vi "_ROSMasterConsole.vi"() -> ()   [LabVIEW 2010]
uses:
  <vilib>/Utility/miscctls.llb/LVRectTypeDef.ctl
  <userlib>/ROSforLV_0.1/ROS/Code/_ROSDefinition.vi
panel:
  in  "Clear Servers?":bool
  in  "expand?":bool
  out "Status":string
  out "Master?":bool
  in  "Tab Control":enum32{"Single Calls", "Servers"}(tab)
  out "TCP Calls":T1(array[cluster])
  out "ROS Master":string="192.168.1.110:11311"
  out "Running?":bool
  out "current task":string
  in  "Stop":bool
  in  "Live Servers":i32(listbox)
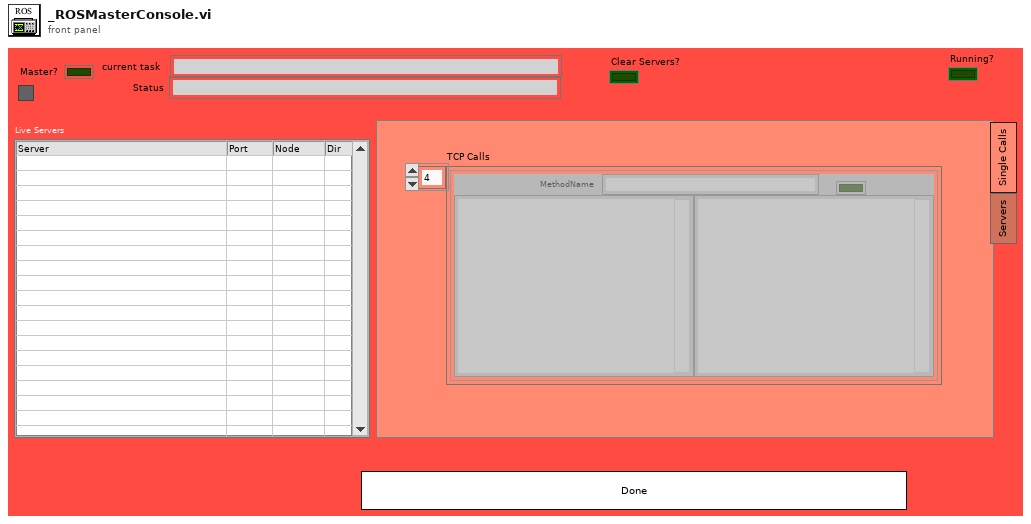
[diagram p1: front panel]
types:
  T1 = cluster{"First":string, "Second":string, "MethodName":string, "success":bool, "Dir1":string, "Dir2":string}[]
  T2 = cluster{"server vi":string, "reference":refnum<vi>, "Description":string[]}[]
  T3 = cluster{"Request":string, "Reply":string, "MethodName":string, "success":bool, "Request 2":string, "Request 3":string}[]
  T4 = cluster{"Request":string, "Reply":string, "MethodName":string, "success":bool, "first string":string, "second string":string}
  T5 = typedef "LVRectTypeDef.ctl" = cluster{"Left":i16, "Top":i16, "Right":i16, "Bottom":i16}
  T6 = typedef "_ROSControl.ctl" = cluster{"topic port":u16, "Node":string, "topic":string, "type":string, "node port":u32, "error ":errorcluster, "Direction":T7, "APIs":string[]}
  T7 = typedef "_ROSDirection.ctl" = enum16{"Node", "Publisher", "Subscriber", "Service Client"}
  T8 = cluster{"server vi":string, "reference":refnum<vi>, "Description":string[]}
  T9 = cluster{"data out":string, "data out 2":string, "data out 3":string, "Success?":bool, "data out 4":string, "data out 5":string}[]
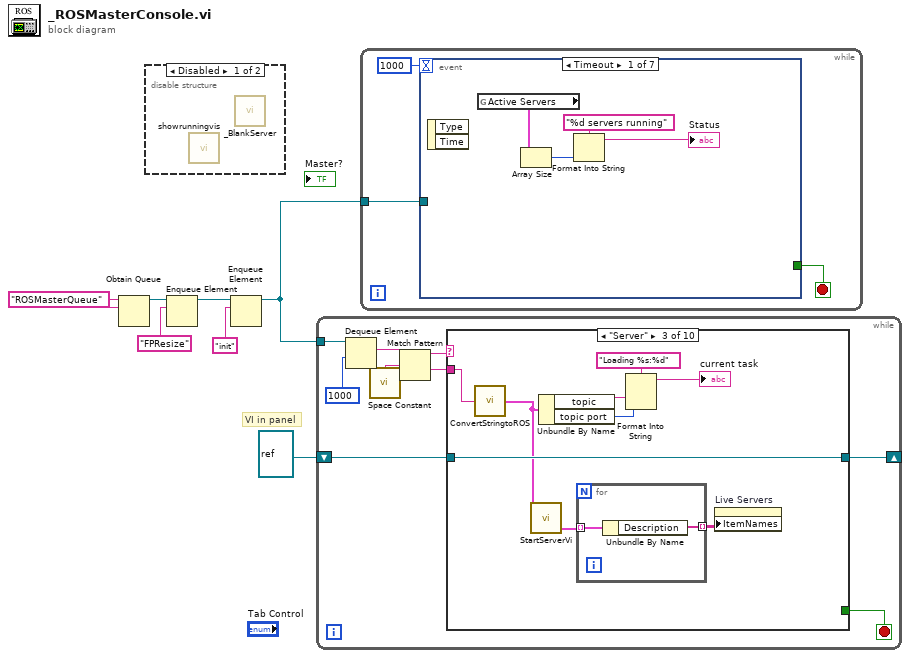
[diagram p0: block diagram]
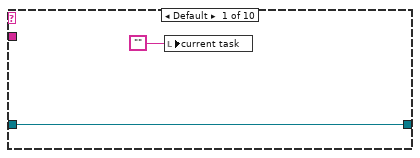
[diagram p3: hidden frame]
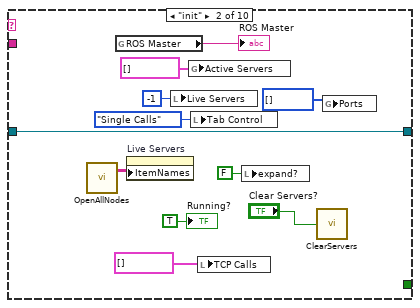
[diagram p4: hidden frame]
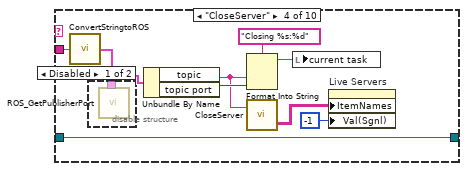
[diagram p5: hidden frame]
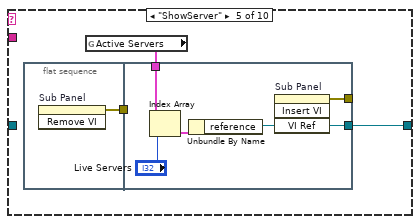
[diagram p7: hidden frame]
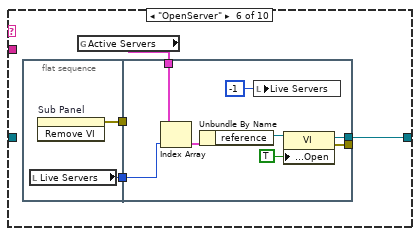
[diagram p8: hidden frame]
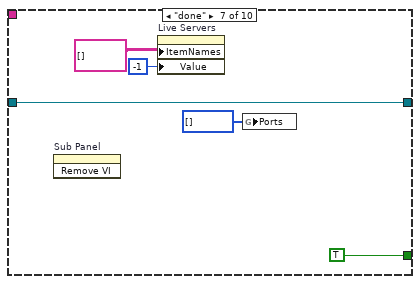
[diagram p9: hidden frame]
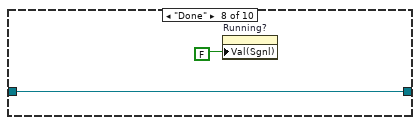
[diagram p10: hidden frame]
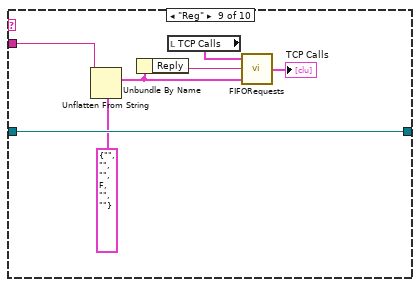
[diagram p11: hidden frame]
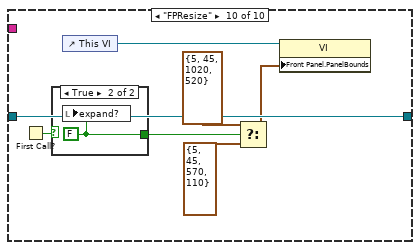
[diagram p12: hidden frame]
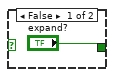
[diagram p13: hidden frame]
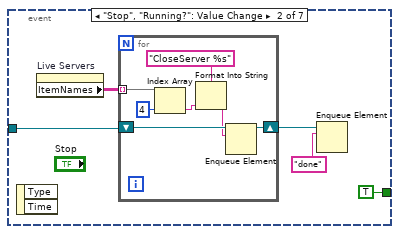
[diagram p14: hidden frame]
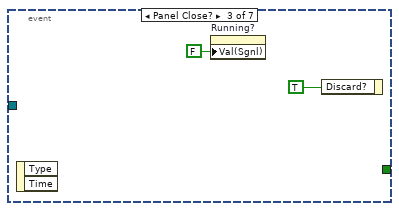
[diagram p15: hidden frame]
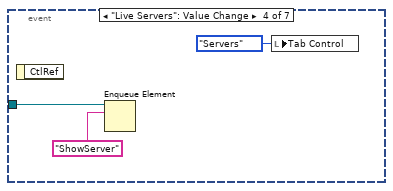
[diagram p16: hidden frame]
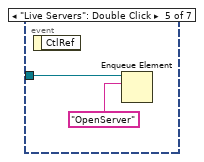
[diagram p17: hidden frame]
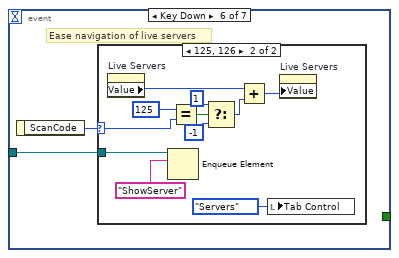
[diagram p18: hidden frame]
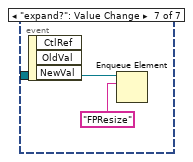
[diagram p20: hidden frame]
diagram:
  w7 = "ROSMasterQueue" ("name (unnamed)")
  # "VI in panel"
  n1 = Obtain Queue(name (unnamed)=w7, element data type=w7) -> (queue out=w4:refnum<queue>)  [unwired: 3 in, 2 out]
  n2 = disable-structure shown="Disabled" {
    frame Disabled {
      n3 = call <userlib>:"showrunningvis.vi"() -> ()  [unwired: 1 in]
      n4 = call <userlib>:"_BlankServer.vi"() -> ()  [unwired: 12 in]
    }
    frame Enabled {
    }
  }
  n5 = Enqueue Element(queue=w4, element="FPResize") -> (queue out=w3:refnum<queue>)  [unwired: 2 in, 2 out]
  n6 = Enqueue Element(queue=w3, element="init") -> (queue out=w6:refnum<queue>)  [unwired: 2 in, 2 out]
  n7 = while {
    tunnel: w6 -> [w16]
    shift-right: [w9] -> _
    shift-left: refnum<vi> refnum ("VI Ref") -> [w10]
    stop <- w15 stop-if-true
    n8 = Dequeue Element(queue=w16, timeout in ms (-1)=1000) -> (element=w13:string)  [unwired: 1 in, 3 out]
    n9 = call <vilib>:"Space Constant.vi"() -> ("String"=w12:string)
    n10 = Match Pattern(string=w13, regular expression=w12) -> (before substring=w14:string, after substring=w11:string)  [unwired: 1 in, 2 out]
    n11 = case shown="\"Server\"" w14 {
      tunnel: [_ _ _ _ _ _ TRUE _ _ _] -> w15
      tunnel: w11 -> [_ _ w35 w44 _ _ _ _ w86 _]
      tunnel: w10 -> [w18 w29 w38 w49 _ _ w77 w80 w87 w94]
      tunnel: [w18 w29 w38 w49 w51 w60 w77 w80 w87 w94] -> w9
      frame Default {
        n12 = local write "current task"("") -> ()
      }
      frame "init" {
        n13 = call <userlib>:"OpenAllNodes.vi"() -> ("Nodes"=w27:string[][])  [unwired: 2 in]
        n14 = global read "_ROSDefinition.vi" "ROS Master"() -> (→"ROS Master":string)
        n15 = property on="Live Servers" class="MCListbox (strict)"("ItemNames"=w27) -> ()  [unwired: 2 in, 2 out]
        n16 = local write "Live Servers"(-1 ("Live Servers")) -> ()
        n17 = global write "_ROSDefinition.vi" "Active Servers"(T2 [] ("Active Servers")) -> ()
        n18 = local write "Tab Control"(enum32{"Single Calls", "Servers"}."Single Calls" ("Tab Control")) -> ()
        n19 = local write "TCP Calls"(T3 [] ("TCP Calls")) -> ()
        n20 = local write "expand?"(FALSE ("expand?")) -> ()
        n21 = call <userlib>:"ClearServers.vi"("Clear Servers?"="Clear Servers?") -> ()  [unwired: 1 out]
        n22 = global write "_ROSDefinition.vi" "Ports"(u16[] [] ("Ports")) -> ()
        "Running?" <- TRUE ("Running?")
      }
      frame "Server" {
        n23 = call <userlib>:"ConvertStringtoROS.vi"("string in"=w35) -> ("ROS"=w31:T6)
        n24 = call <userlib>:"StartServerVi.vi"("Baxter"=w31) -> ("Active Topics"=w32:T2)  [unwired: 2 out]
        n25 = Unbundle By Name(w31) -> ("topic"=w34:string, "topic port"=w33:u16)
        n26 = for {
          tunnel: w32 -> [w40] mode=indexing
          tunnel: [w39] -> w30 mode=indexing
          n27 = Unbundle By Name(w40) -> ("Description"=w39:string[])
        }
        n28 = Format Into String(format string="Loading %s:%d", w34, w33) -> (resulting string=→"current task":string)  [unwired: 2 in, 1 out]
        n29 = property on="Live Servers" class="MCListbox (strict)"("ItemNames"=w30) -> ()  [unwired: 2 in, 2 out]
      }
      frame "CloseServer" {
        n30 = call <userlib>:"ConvertStringtoROS.vi"("string in"=w44) -> ("ROS"=w41:T6)
        n31 = disable-structure shown="Disabled" {
          disable-tunnel: w41 -> [w50 _]
          frame Disabled {
            n32 = call <userlib>:"ROS_GetPublisherPort.vi"("ROS in"=w50) -> ()  [unwired: 1 in, 2 out]
          }
          frame Enabled {
          }
        }
        n33 = Unbundle By Name(w41) -> ("topic"=w42:string, "topic port"=w43:u16)
        n34 = Format Into String(format string="Closing %s:%d", w42, w43) -> (resulting string=w47:string)  [unwired: 2 in, 1 out]
        n35 = call <userlib>:"CloseServer.vi"("Server"=w42) -> ("Active Servers Out"=w46:string[][])  [unwired: 2 in]
        n36 = local write "current task"(w47) -> ()
        n37 = property on="Live Servers" class="MCListbox (strict)"("ItemNames"=w46, "Val(Sgnl)"=-1 ("Value (Signaling)")) -> ()  [unwired: 2 in, 2 out]
      }
      frame "ShowServer" {
        n38 = flat-sequence {
          tunnel: [w54] -> w53
          tunnel: w53 -> [_]
          tunnel: [w58] -> _
          tunnel: w52 -> [w57]
          tunnel: [w55] -> w51
          frame #0 {
            n39 = invoke on="Sub Panel" class="SubPanel" method="Remove VI"() -> (error out=w54:errorcluster)  [unwired: 3 in, 2 out]
          }
          frame #1 {
            n40 = Index Array(array=w57, index="Live Servers") -> (element=w56:T8)
            n41 = Unbundle By Name(w56) -> ("reference"=w55:refnum<vi>)
            n42 = invoke on="Sub Panel" class="SubPanel" method="Insert VI"("VI Ref"=w55) -> (error out=w58:errorcluster)  [unwired: 3 in, 3 out]
          }
        }
        n43 = global read "_ROSDefinition.vi" "Active Servers"() -> (w52:T2)
      }
      frame "OpenServer" {
        n44 = flat-sequence {
          tunnel: [w65] -> w63
          tunnel: [w64] -> w62
          tunnel: w63 -> [_]
          tunnel: w62 -> [w72]
          tunnel: w61 -> [w70]
          tunnel: [w67] -> w60
          tunnel: [w66] -> _
          frame #0 {
            n45 = local read "Live Servers"() -> (w64:i32)
            n46 = invoke on="Sub Panel" class="SubPanel" method="Remove VI"() -> (error out=w65:errorcluster)  [unwired: 3 in, 2 out]
          }
          frame #1 {
            n47 = Index Array(array=w70, index=w72) -> (element=w69:T8)
            n48 = Unbundle By Name(w69) -> ("reference"=w68:refnum<vi>)
            n49 = local write "Live Servers"(-1 ("Live Servers")) -> ()
            n50 = property class="VI"(reference=w68, "Front Panel.Open"=TRUE ("Front Panel Window:Open")) -> (reference out=w67:refnum<vi>, error out=w66:errorcluster)  [unwired: 1 in]
          }
        }
        n51 = global read "_ROSDefinition.vi" "Active Servers"() -> (w61:T2)
      }
      frame "done" {
        n52 = invoke on="Sub Panel" class="SubPanel" method="Remove VI"() -> ()  [unwired: 3 in, 3 out]
        n53 = property on="Live Servers" class="MCListbox (strict)"("ItemNames"=string[][] [] ("Item Names"), "Value"=-1 ("Live Servers")) -> ()  [unwired: 2 in, 2 out]
        n54 = global write "_ROSDefinition.vi" "Ports"(u16[] [] ("Ports")) -> ()
      }
      frame "Done" {
        n55 = property on="Running?" class="Bool (strict)"("Val(Sgnl)"=FALSE) -> ()  [unwired: 2 in, 2 out]
      }
      frame "Reg" {
        n56 = Unflatten From String(type=T4 {"Request"="", "Reply"="", "MethodName"="", "success"=FALSE, "first string"="", "second string"=""} ("Reg"), binary string=w86) -> (value=w82:T4)  [unwired: 3 in, 2 out]
        n57 = Unbundle By Name(w82) -> ("Reply"=w81:string)
        n58 = local read "TCP Calls"() -> (w84:T1)
        n59 = call <userlib>:"FIFORequests.vi"("New One"=w82, "data out"=w81, "Requests In"=w84) -> ("Requests Out"=→"TCP Calls":T9)
      }
      frame "FPResize" {
        n60 = First Call?() -> (First Call?: T/F=w89:bool)
        n61 = case shown="True" w89 {
          tunnel: ["expand?" w96] -> w88
          frame False {
          }
          frame True {
            w96 = FALSE ("expand?")
            n62 = local write "expand?"(w96) -> ()
          }
        }
        n63 = control-ref of="This VI"() -> (w93:refnum<vi>)
        n64 = Select(t=T5 {"Left"=5, "Top"=45, "Right"=1020, "Bottom"=520} ("Front Panel Window:Panel Bounds"), s=w88, f=T5 {"Left"=5, "Top"=45, "Right"=570, "Bottom"=110} ("Front Panel Window:Panel Bounds")) -> (s? t:f=w91:T5)
        n65 = property class="VI"(reference=w93, "Front Panel.PanelBounds"=w91) -> ()  [unwired: 1 in, 2 out]
      }
    }
  }
  n66 = while {
    tunnel: w6 -> [w99]
    stop <- w98 stop-if-true
    n67 = event shown="[0] Timeout" {
      selector: _ -> [_ _ _ _ _ _ _]
      dyn-events: _ -> [_ _ _ _ _ _ _]
      timeout: 1000 -> [_ _ _ _ _ _ _]
      tunnel: w99 -> [_ w106 _ w119 w121 w124 w136]
      tunnel: [_ TRUE ("Stop") _ _ _ _ _] -> w98
      event Timeout {
        n68 = event-data() -> ()  [unwired: 1 in, 2 out]
        n69 = global read "_ROSDefinition.vi" "Active Servers"() -> (w100:T2)
        n70 = Array Size(array=w100) -> (size(s)=w103:i32)
        n71 = Format Into String(format string="%d servers running", w103) -> (resulting string=→"Status":string)  [unwired: 2 in, 1 out]
      }
      event "Stop", "Running?": Value Change {
        n72 = event-data() -> ()  [unwired: 1 in, 2 out]
        n73 = property on="Live Servers" class="MCListbox (strict)"() -> ("ItemNames"=w107:string[][])  [unwired: 2 in, 2 out]
        n74 = for {
          tunnel: w107 -> [w115] mode=indexing
          shift-right: [w109] -> w105
          shift-left: w106 -> [w111]
          n75 = Index Array(array=w115, index=4) -> (element=w113:string)
          n76 = Format Into String(format string="CloseServer %s", w113) -> (resulting string=w110:string)  [unwired: 2 in, 1 out]
          n77 = Enqueue Element(queue=w111, element=w110) -> (queue out=w109:refnum<queue>)  [unwired: 2 in, 2 out]
        }
        n78 = Enqueue Element(queue=w105, element="done") -> ()  [unwired: 2 in, 3 out]
      }
      event Panel Close? {
        n79 = event-data() -> ()  [unwired: 1 in, 2 out]
        n80 = property on="Running?" class="Bool (strict)"("Val(Sgnl)"=FALSE ("Value (Signaling)")) -> ()  [unwired: 2 in, 2 out]
        n81 = event-data("Discard?"=TRUE ("Stop")) -> ()  [unwired: 1 in, 1 out]
      }
      event "Live Servers": Value Change {
        n82 = event-data() -> ()  [unwired: 1 in, 1 out]
        n83 = Enqueue Element(queue=w119, element="ShowServer") -> ()  [unwired: 2 in, 3 out]
        n84 = local write "Tab Control"(enum32{"Single Calls", "Servers"}."Servers" ("Tab Control")) -> ()
      }
      event "Live Servers": Double Click {
        n85 = event-data() -> ()  [unwired: 1 in, 1 out]
        n86 = Enqueue Element(queue=w121, element="OpenServer") -> ()  [unwired: 2 in, 3 out]
      }
      event Key Down {
        # "Ease navigation of live servers"
        n87 = event-data() -> ("ScanCode"=w123:i16)  [unwired: 1 in]
        n88 = case shown="125, 126" w123 {
          selector: w123 -> [_ w132]
          tunnel: w124 -> [_ w135]
          frame Default {
          }
          frame 125, 126 {
            n89 = property on="Live Servers" class="MCListbox (strict)"() -> ("Value"=w128:i32)  [unwired: 2 in, 2 out]
            n90 = Enqueue Element(queue=w135, element="ShowServer") -> ()  [unwired: 2 in, 3 out]
            n91 = Equal?(x=i16 125, y=w132) -> (x = y?=w130:bool)
            n92 = Select(t=i16 1 ("x"), s=w130, f=i16 -1 ("x")) -> (s? t:f=w127:i16)
            n93 = Add(x=w128, y=w127) -> (x+y=w129:i32)
            n94 = local write "Tab Control"(enum32{"Single Calls", "Servers"}."Servers" ("Tab Control")) -> ()
            n95 = property on="Live Servers" class="MCListbox (strict)"("Value"=w129) -> ()  [unwired: 2 in, 2 out]
          }
        }
      }
      event "expand?": Value Change {
        n96 = event-data() -> ()  [unwired: 1 in, 3 out]
        n97 = Enqueue Element(queue=w136, element="FPResize") -> ()  [unwired: 2 in, 3 out]
      }
    }
  }
